vi "CreateObjects__slk_mt.vi"(8 "error in (no error)":errorcluster, 11 "control refnums in":refnum<vi>[](array[refnum])) -> (0 "error out":errorcluster, 3 "objects out":refnum<class "GUI__slk_mt.lvclass">[](array[class]))   [LabVIEW 2013, in "Lazyboots Menu Tool.lvlib"]
doc: "Creates object by control refnums.\n\nThis is a specification design pattern for dynamic dispatching. Adding a new case frame when add a new data type on <b>Options</b> GUI."
uses:
  Library/Lazyboots Menu Tool.lvlib
  Class/GUI/GUI__slk_mt.lvclass
  Class/Boolean/Boolean__slk_mt.lvclass
  Class/Digital U32/Digital U32__slk_mt.lvclass
  Class/ComboBox/ComboBox__slk_mt.lvclass
  Class/Ring/Ring__slk_mt.lvclass
panel:
  # "CreateObjects__slk_mt.vi\nCreates object by control refnums.\n\nNOTICE -- YOU MUST LEAVE THIS NOTICE IN PLACE.\n\nCopyright (c) 2011, LIANG LIU Shawn.Liu.cn@gmail.com\nAll rights reserved.\n\nRedistribution and use in source and binary forms, with or without modification, are permitted provided that the following conditions are met:\n-Redistributions of source code must retain the above copyright notice, this list of conditions and the following disclaimer.\n-Redistributions in binary form must reproduce the above copyright notice, this list of conditions and the following disclaimer in the documentation and/or other materials provided with the distribution.\n-Neither the name of the eLp nor the names of its contributors may be used to endorse or promote products derived from this software without specific prior written permission.\n\nTHIS SOFTWARE IS PROVIDED BY THE COPYRIGHT HOLDERS AND CONTRIBUTORS \"AS IS\" AND ANY EXPRESS OR IMPLIED WARRANTIES, INCLUDING, BUT NOT LIMITED TO, THE IMPLIED WARRANTIES OF MERCHANTABILITY AND FITNESS FOR A PARTICULAR PURPOSE ARE DISCLAIMED. IN NO EVENT SHALL THE COPYRIGHT HOLDER OR CONTRIBUTORS BE LIABLE FOR ANY DIRECT, INDIRECT, INCIDENTAL, SPECIAL, EXEMPLARY, OR CONSEQUENTIAL DAMAGES (INCLUDING, BUT NOT LIMITED TO, PROCUREMENT OF SUBSTITUTE GOODS OR SERVICES; LOSS OF USE, DATA, OR PROFITS; OR BUSINESS INTERRUPTION) HOWEVER CAUSED AND ON ANY THEORY OF LIABILITY, WHETHER IN CONTRACT, STRICT LIABILITY, OR TORT (INCLUDING NEGLIGENCE OR OTHERWISE) ARISING IN ANY WAY OUT OF THE USE OF THIS SOFTWARE, EVEN IF ADVISED OF THE POSSIBILITY OF SUCH DAMAGE."
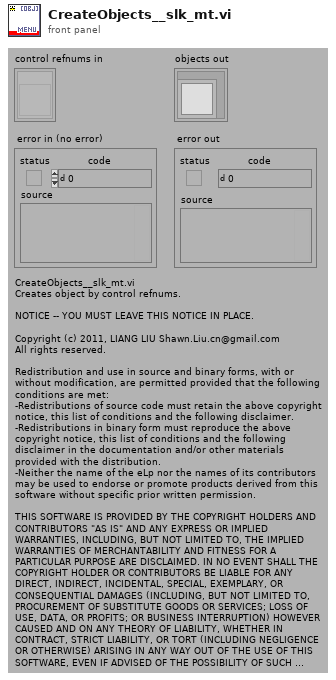
[diagram p1: front panel]
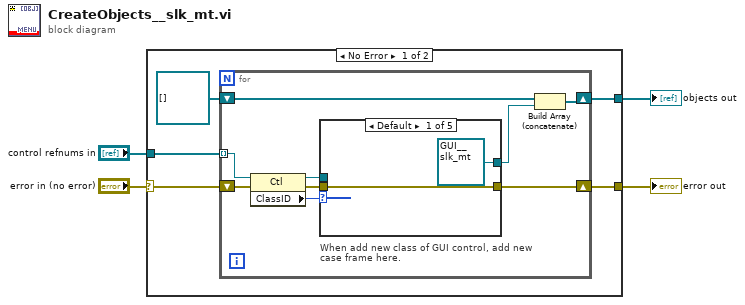
[diagram p0: block diagram]
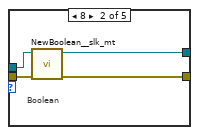
[diagram p2: hidden frame]
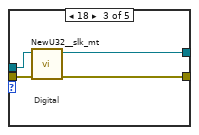
[diagram p3: hidden frame]
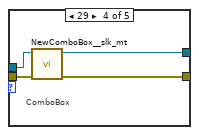
[diagram p4: hidden frame]
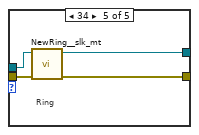
[diagram p5: hidden frame]
diagram:
  n1 = case shown="No Error" "error in (no error)" {
    selector: "error in (no error)" -> [w5 w37]
    tunnel: "control refnums in" -> [w8 _]
    tunnel: [w7 _] -> w3
    tunnel: [w6 w37] -> w2
    frame No Error {
      n2 = for {
        shift-right: [w13] -> w7
        shift-left: refnum<class "GUI__slk_mt.lvclass">[] [] ("Objects") -> [w14]
        tunnel: w8 -> [w11] mode=indexing
        shift-right: [w15] -> w6
        shift-left: w5 -> [w18]
        n3 = property class="Ctl"(reference=w11, error in=w18) -> (reference out=w10:refnum<vi>, error out=w16:errorcluster, "ClassID"=w17:u32)
        n4 = case "When add new class of GUI control, add new case frame here." shown="Default" w17 {
          tunnel: w16 -> [w20 w24 w28 w32 w36]
          tunnel: [w20 w23 w27 w31 w35] -> w15
          tunnel: [refnum<class "GUI__slk_mt.lvclass"> refnum ("digital u32__slk_mt out") w22 w26 w30 w34] -> w12
          tunnel: w10 -> [_ w21 w25 w29 w33]
          frame Default {
          }
          frame 8 {
            # "Boolean"
            n5 = call "NewBoolean__slk_mt.vi"("error in (no error)"=w24, "control refnum in"=w21) -> ("error out"=w23:errorcluster, "boolean out"=w22:refnum<class "Boolean__slk_mt.lvclass">)  [unwired: 8 in]
          }
          frame 18 {
            # "Digital"
            n6 = call "NewU32__slk_mt.vi"("error in (no error)"=w28, "control refnum in"=w25) -> ("error out"=w27:errorcluster, "digital u32 out"=w26:refnum<class "Digital U32__slk_mt.lvclass">)  [unwired: 8 in]
          }
          frame 29 {
            # "ComboBox"
            n7 = call "NewComboBox__slk_mt.vi"("error in (no error)"=w32, "control refnum in"=w29) -> ("error out"=w31:errorcluster, "combobox out"=w30:refnum<class "ComboBox__slk_mt.lvclass">)  [unwired: 8 in]
          }
          frame 34 {
            # "Ring"
            n8 = call "NewRing__slk_mt.vi"("error in (no error)"=w36, "control refnum in"=w33) -> ("error out"=w35:errorcluster, "ring out"=w34:refnum<class "Ring__slk_mt.lvclass">)  [unwired: 8 in]
          }
        }
        n9 = Build Array (concatenate)(w14, w12) -> (w13:refnum<class "GUI__slk_mt.lvclass">[])
      }
    }
    frame Error {
    }
  }
  "objects out" <- w3
  "error out" <- w2
